vi "Get plot length.vi"(2 "Max phase":dbl, 3 "Plot length scale":dbl format="%#_13g", 4 "Plot length (min)":dbl format="%#_13g") -> (0 "New plot length scale":dbl, 1 "New plot length":dbl)   [LabVIEW 2020]
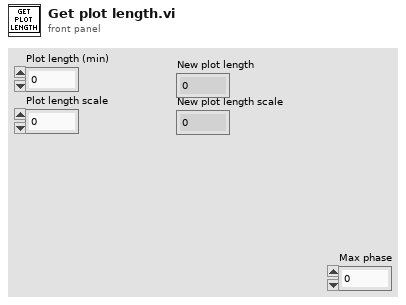
[diagram p1: front panel]
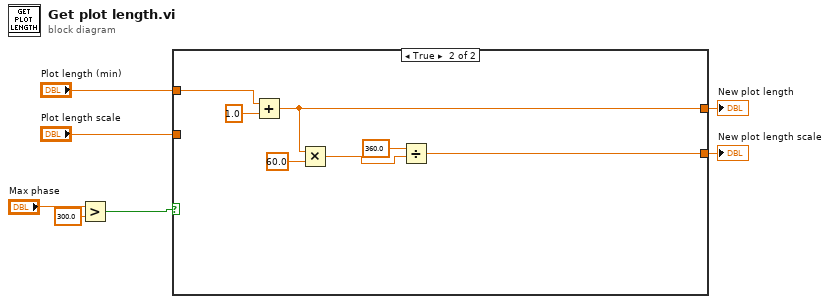
[diagram p0: block diagram]
diagram:
  n1 = Greater?(x="Max phase", y=300.0) -> (0:w5:bool)
  n2 = case shown="True" w5 {
    tunnel: "Plot length (min)" -> [w9 w16]
    tunnel: [w9 w13] -> w1
    tunnel: [w8 w10] -> w2
    tunnel: "Plot length scale" -> [w8 _]
    frame False {
    }
    frame True {
      n3 = Add(x=w16, y=1.0) -> (x+y=w13:dbl)
      n4 = Multiply(x=w13, y=60.0) -> (x*y=w11:dbl)
      n5 = Divide(x=360.0, y=w11) -> (x/y=w10:dbl)
    }
  }
  "New plot length scale" <- w2
  "New plot length" <- w1
